vi "Internal Components.vi"(8 "error in (no error)":errorcluster) -> (0 "error out":errorcluster, 3 "Components":refnum<class "Component.lvclass">[](array[class]))   [LabVIEW 2017, in "DSF Core.lvlib"]
uses:
  DSF Core.lvlib
  Component/Component.lvclass
  Components/Buffer Converters/DSF Type Converter/DSF Buffer Converter.lvclass
  Components/Transceivers/UDP/UDP Transceiver.lvclass
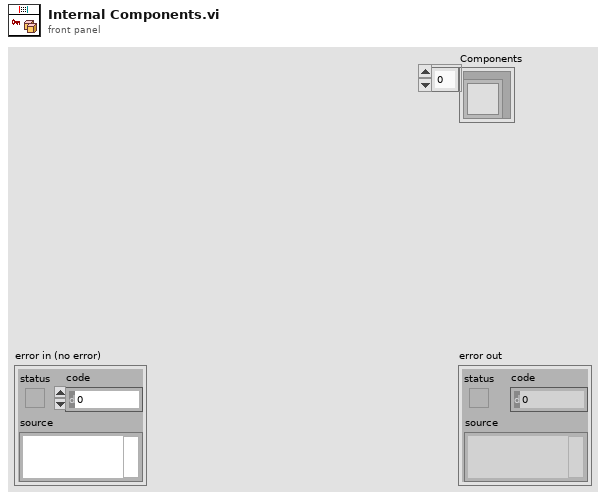
[diagram p1: front panel]
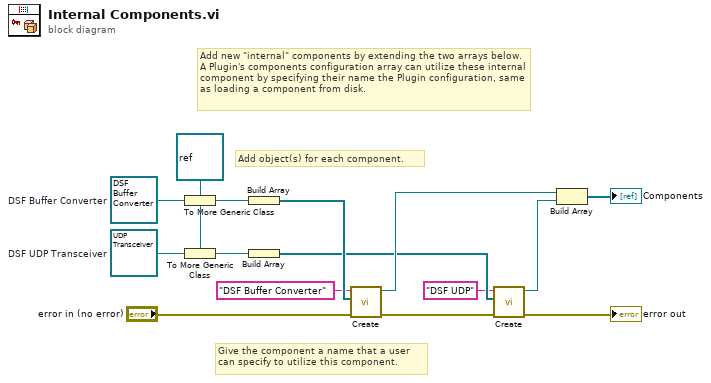
[diagram p0: block diagram]
diagram:
  w14 = refnum<class "UDP Transceiver.lvclass"> refnum  # DSF UDP Transceiver
  w13 = refnum<class> refnum ("LabVIEW Object")
  w15 = refnum<class "DSF Buffer Converter.lvclass"> refnum  # DSF Buffer Converter
  # "Give the component a name that a user can specify to utilize this component."
  # "Add object(s) for each component."
  # "Add new \"internal\" components by extending the two arrays below. A Plugin's components configuration array can utilize these internal component by specifying their name the Plugin configuration, same as loading a component from disk."
  n1 = To More Generic Class(target class=w13, reference=w15) -> (generic class reference=w12:refnum<class>)
  n2 = To More Generic Class(target class=w13, reference=w14) -> (generic class reference=w7:refnum<class>)
  n3 = Build Array(w12) -> (w11:refnum<class>[])
  n4 = Build Array(w7) -> (w6:refnum<class>[])
  n5 = call "Create.vi"("error in (no error)"="error in (no error)", "objects"=w11, "name"="DSF Buffer Converter") -> ("error out"=w2:errorcluster, "Component"=w10:refnum<class "Component.lvclass">)  [unwired: 7 in]
  n6 = call "Create.vi"("error in (no error)"=w2, "objects"=w6, "name"="DSF UDP") -> ("error out"=→"error out":errorcluster, "Component"=w9:refnum<class "Component.lvclass">)  [unwired: 7 in]
  n7 = Build Array(w10, w9) -> (→"Components":refnum<class "Component.lvclass">[])
